vi "Absolute.vi"(10 "Path in":path) -> (2 "Path out":path)   [LabVIEW 2022 SP3, in "PathUtils.lvlib"]
uses:
  PathUtils.lvlib
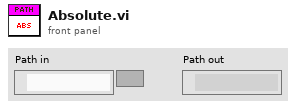
[diagram p1: front panel]
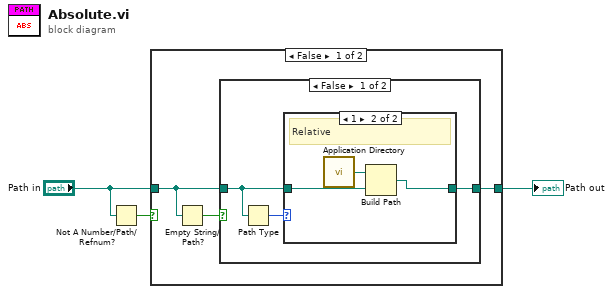
[diagram p0: block diagram]
diagram:
  n1 = Not A Number/Path/Refnum?(number/path/refnum="Path in") -> (NaN/Path/Refnum?=w2:bool)
  n2 = case shown="False" w2 {
    tunnel: [w5 w15] -> w3
    tunnel: "Path in" -> [w4 w15]
    frame False {
      n3 = Empty String/Path?(string/path=w4) -> (empty?=w6:bool)
      n4 = case shown="False" w6 {
        tunnel: w4 -> [w7 w14]
        tunnel: [w8 w14] -> w5
        frame False {
          n5 = Path Type(1:w7) -> (0:w9:i16)
          n6 = case shown="1" w9 {
            tunnel: [w10 w11] -> w8
            tunnel: w7 -> [w10 w12]
            frame 0, Default {
              # "Absolute"
            }
            frame 1 {
              # "Relative"
              n7 = call <vilib>:"Application Directory.vi"() -> ("Application Directory"=w13:path)
              n8 = Build Path(base path=w13, name or relative path=w12) -> (appended path=w11:path)
            }
          }
        }
        frame True {
        }
      }
    }
    frame True {
    }
  }
  "Path out" <- w3
